vi "TIMEOUT_CONNECT_TO_BOARD.vi"(11 "TIMEBEGIN":u32) -> (1 "STATUS":bool, 3 "TIMEOUT":u32)   [LabVIEW 2017]
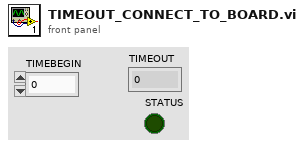
[diagram p1: front panel]
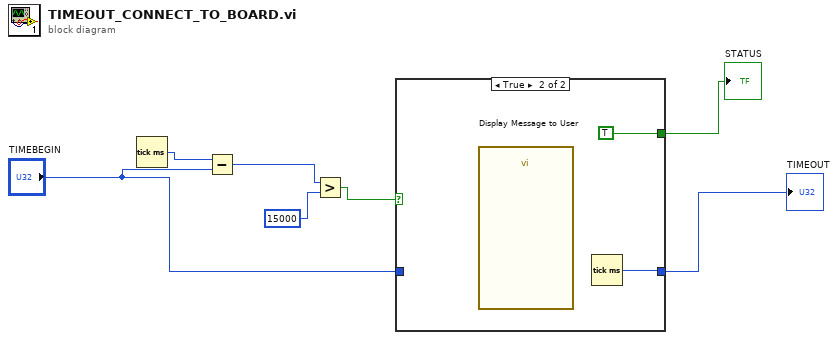
[diagram p0: block diagram]
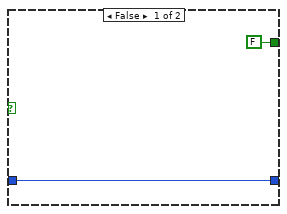
[diagram p2: hidden frame]
diagram:
  n1 = Tick Count (ms)() -> (millisecond timer value=w7:u32)
  n2 = Subtract(x=w7, y="TIMEBEGIN") -> (x-y=w6:u32)
  n3 = Greater?(x=w6, y=u32 15000) -> (0:w4:bool)
  n4 = case shown="True" w4 {
    tunnel: [w9 w11] -> w3
    tunnel: "TIMEBEGIN" -> [w9 _]
    tunnel: [FALSE ("STATUS") TRUE ("STATUS")] -> w1
    frame False {
    }
    frame True {
      n5 = call "Display Message to User"() -> ()  [unwired: 10 in, 2 out]
      n6 = Tick Count (ms)() -> (millisecond timer value=w11:u32)
    }
  }
  "TIMEOUT" <- w3
  "STATUS" <- w1
